vi "fake_read_from_fifo.vi"(7 "fakeJust1and0":bool, 9 "acquire":bool, 11 "iteration counter":u16) -> (0 "num fake pixels read":u32, 1 "num fake fifo timeouts":u32, 3 "fake photons":T1)   [LabVIEW 2010]
uses:
  common_typedefs/channels_cluster.ctl
  <vilib>/rvi/DataTransferAndStorage/Container/XNode/niFpgaContainer.xnode
  <vilib>/rvi/DataTransferAndStorage/Container/Common/niFpgaContainerMethod.ctl
  <vilib>/rvi/DataTransferAndStorage/Container/Common/niFpgaTransferTypeControl.ctl
  <vilib>/rvi/interface/RandomDataEmulation/nirviRandomDataFPGAFIFO.vi
  <vilib>/rvi/interface/RandomDataEmulation/niFpgaRandomDataHandleErrors.vi
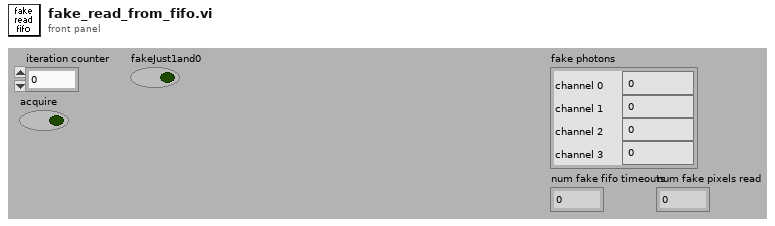
[diagram p1: front panel]
types:
  T1 = typedef "channels_cluster.ctl" = cluster{"channel 0":u32, "channel 1":u32, "channel 2":u32, "channel 3":u32}
  T2 = typedef "niFpgaContainerMethod.ctl" = enum16{"<none>", "write", "read", "clear", "getNumberOfElementsToWrite", "getNumberOfElementsToRead", "enable", "disable", "flushAndDisable", "getStreamState", "readA", "readB", "dramWrite", "dramWriteWithByteEnables", "dramRequestData", "dramRetrieveData"}
  T3 = typedef "niFpgaTransferTypeControl.ctl" = enum16{"Target-Scoped", "Host to Target - DMA", "Target to Host - DMA", "Peer to Peer Reader", "Peer to Peer Writer", "Bidirectional"}
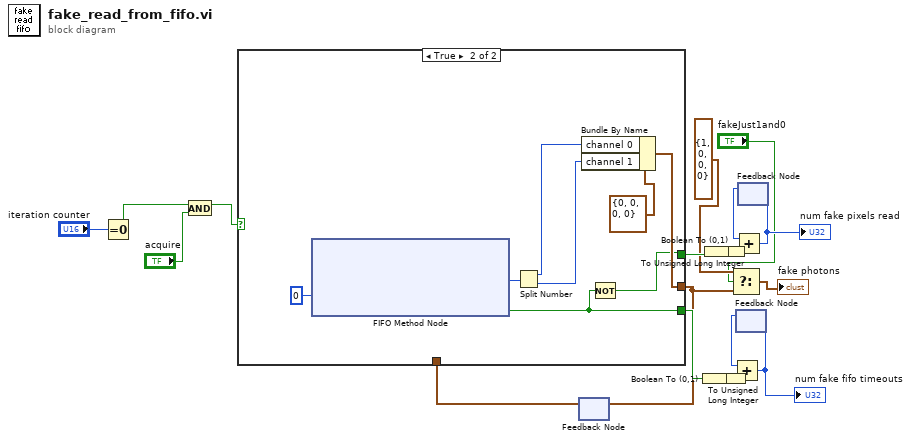
[diagram p0: block diagram]
diagram:
  n1 = Equal To 0?(x="iteration counter") -> (x = 0?=w1:bool)
  n2 = And(x=w1, y="acquire") -> (x .and. y?=w13:bool)
  n3 = feedback #1() -> (w18:T1)  [unwired: 1 in]
  n4 = case shown="True" w13 {
    tunnel: [w20 w27] -> w5
    tunnel: w18 -> [w20 _]
    tunnel: [_ w22] -> w8
    tunnel: [_ w21] -> w17
    frame False {
    }
    frame True {
      n5 = xnode ("FIFO Method Node")("Timeout"=0) -> ("Element"=w25:u32, "Timed Out?"=w22:bool)  [unwired: 1 in, 1 out]
      n6 = Split Number(x=w25) -> (hi(x)=w24:u16, lo(x)=w23:u16)
      n7 = Bundle By Name(cluster=T1 {"channel 0"=0, "channel 1"=0, "channel 2"=0, "channel 3"=0} ("input cluster"), "channel 0"=w24, "channel 1"=w23) -> (w27:T1)
      n8 = Not(x=w22) -> (.not. x?=w21:bool)
    }
  }
  n9 = feedback-in #1(w5) -> ()
  n10 = Boolean To (0,1)(Boolean=w8) -> (0, 1=w11:i16)
  n11 = Boolean To (0,1)(Boolean=w17) -> (0, 1=w16:i16)
  n12 = To Unsigned Long Integer(number=w16) -> (unsigned 32bit integer=w7:u32)
  n13 = To Unsigned Long Integer(number=w11) -> (unsigned 32bit integer=w6:u32)
  n14 = Select(t=T1 {"channel 0"=1, "channel 1"=0, "channel 2"=0, "channel 3"=0}, s="fakeJust1and0", f=w5) -> (s? t:f=→"fake photons":T1)
  n15 = feedback #2() -> (w9:u32)  [unwired: 1 in]
  n16 = Add(x=w9, y=w6) -> (x+y=w10:u32)
  "num fake fifo timeouts" <- w10
  n17 = feedback-in #2(w10) -> ()
  n18 = feedback #3() -> (w14:u32)  [unwired: 1 in]
  n19 = Add(x=w14, y=w7) -> (x+y=w15:u32)
  "num fake pixels read" <- w15
  n20 = feedback-in #3(w15) -> ()
